vi "Misc.vi"() -> ()   [LabVIEW 2017]
panel:
  out "check":dbl=200.0
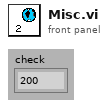
[diagram p1: front panel]
diagram:
